vi "Limits.vi"(5 "Y Max":dbl=nan, 7 "Y Min":dbl=nan, 8 "error in (no error)":errorcluster, 9 "X Max":dbl=nan, 10 "X Min":dbl=nan, 11 "Plot ID":T1 format="%x") -> (0 "error out":errorcluster, 3 "Plot ID Out":T1 format="%x")   [LabVIEW 2013, in "Advanced Plotting Toolkit.lvlib"]
doc: "Set ranges for the X and Y axes. All inputs are optional."
uses:
  Advanced Plotting Toolkit.lvlib
  typedefs/PlotID.ctl
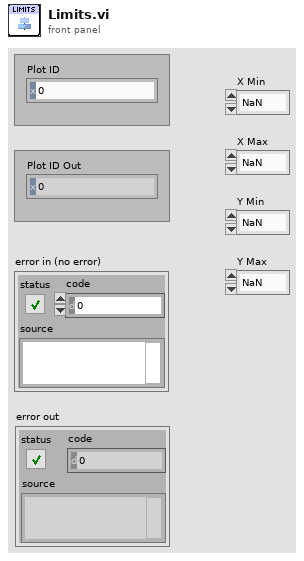
[diagram p1: front panel]
types:
  T1 = typedef "Advanced Plotting Toolkit.lvlib/PlotID.ctl" = i32
  T2 = typedef "Advanced Plotting Toolkit.lvlib/KeyValue.ctl" = cluster{"Key":string, "Value":string}
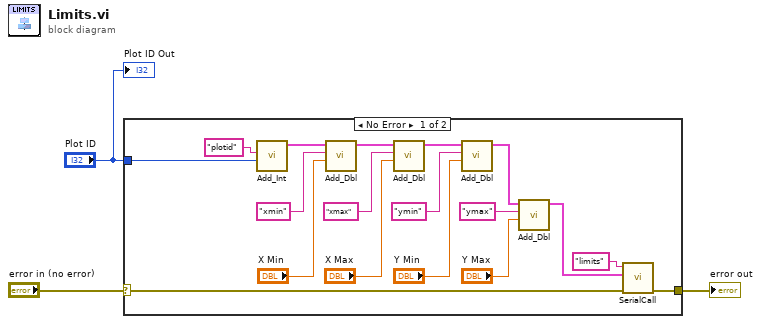
[diagram p0: block diagram]
diagram:
  n1 = case shown="No Error" "error in (no error)" {
    selector: "error in (no error)" -> [w5 w22]
    tunnel: "Plot ID" -> [w8 _]
    tunnel: [w4 w22] -> w1
    frame No Error {
      n2 = call "Add_Int.vi"("Value"=w8, "Key"="plotid") -> ("Keyword Array Out"=w16:T2[])  [unwired: 9 in]
      n3 = call "Add_Dbl.vi"("Value"="X Min", "Key"="xmin", "Keyword Array"=w16) -> ("Keyword Array Out"=w15:T2[])  [unwired: 8 in]
      n4 = call "Add_Dbl.vi"("Value"="X Max", "Key"="xmax", "Keyword Array"=w15) -> ("Keyword Array Out"=w14:T2[])  [unwired: 8 in]
      n5 = call "Add_Dbl.vi"("Value"="Y Min", "Key"="ymin", "Keyword Array"=w14) -> ("Keyword Array Out"=w13:T2[])  [unwired: 8 in]
      n6 = call "Add_Dbl.vi"("Value"="Y Max", "Key"="ymax", "Keyword Array"=w13) -> ("Keyword Array Out"=w7:T2[])  [unwired: 8 in]
      n7 = call "SerialCall.vi"("error in (no error)"=w5, "data"=w7, "Resource"="limits") -> ("error out"=w4:errorcluster)  [unwired: 7 in, 1 out]
    }
    frame Error {
    }
  }
  "error out" <- w1
  "Plot ID Out" <- "Plot ID"
